vi "User32dllAPI.FindWindow.vi"(8 "error in (no error)":errorcluster, 10 "WindowName":string) -> (0 "error out":errorcluster, 3 "hWnd":i32)   [LabVIEW 2019, in "Tools.lvlib"]
uses:
  Tools.lvlib
  user32.dll
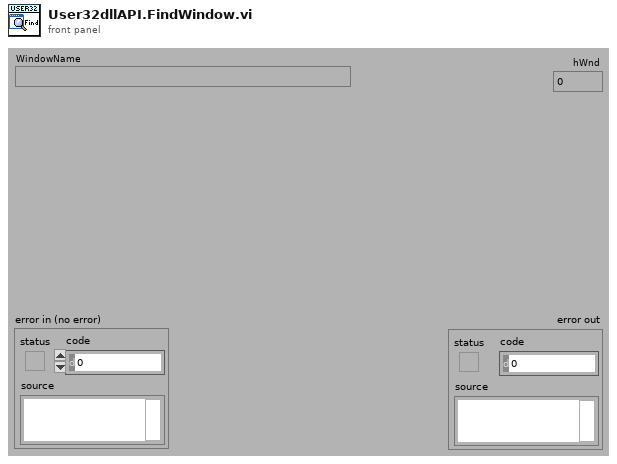
[diagram p1: front panel]
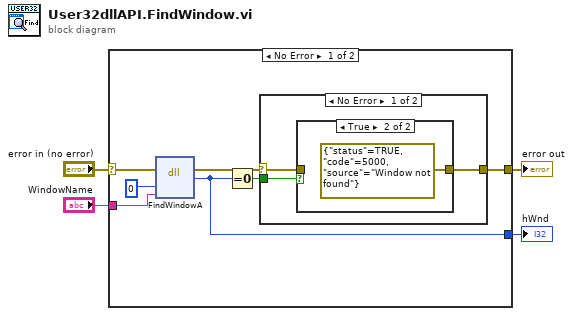
[diagram p0: block diagram]
diagram:
  n1 = case shown="No Error" "error in (no error)" {
    selector: "error in (no error)" -> [w10 w18]
    tunnel: [w8 w18] -> w2
    tunnel: [w7 _] -> w3
    tunnel: "WindowName" -> [w6 _]
    frame No Error {
      n2 = dll-call lib="USER32.DLL" fn="FindWindowA"(error in=w10, "lpClassName"=0, "lpWindowName"=w6) -> (error out=w9:errorcluster, "hWnd"=w7:i32)  [unwired: 4 in, 1 out]
      n3 = Equal To 0?(x=w7) -> (x = 0?=w11:bool)
      n4 = case shown="No Error" w9 {
        selector: w9 -> [w12 w17]
        tunnel: w11 -> [w14 _]
        tunnel: [w13 w17] -> w8
        frame No Error {
          n5 = case shown="True" w14 {
            tunnel: [w15 errorcluster {"status"=TRUE, "code"=5000, "source"="Window not found"} ("error out")] -> w13
            tunnel: w12 -> [w15 _]
            frame False {
            }
            frame True {
            }
          }
        }
        frame Error {
        }
      }
    }
    frame Error {
    }
  }
  "hWnd" <- w3
  "error out" <- w2
